vi "Monitor temp.vi"(8 "error in (no error)":errorcluster, 10 "Address":dbl=1.0, 11 "VISA resource name (IN)":refnum<visa-resource-name>) -> (0 "error out":errorcluster, 2 "Recevied Temp.  data":dbl, 3 "VISA resource name (OUT)":refnum<visa-resource-name>)   [LabVIEW 2010, in "Yudian AI508.lvlib"]
doc: "Use this template to build a VI to use as a subVI."
uses:
  <instrlib>/Yudian AI508/Yudian AI508.lvlib
panel:
  out "Recieved Raw Data":string
  out "Data buffer":string
  out "Digital shift":i32
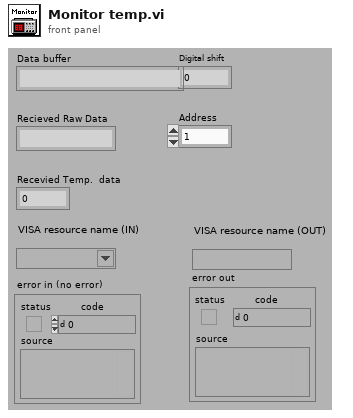
[diagram p1: front panel]
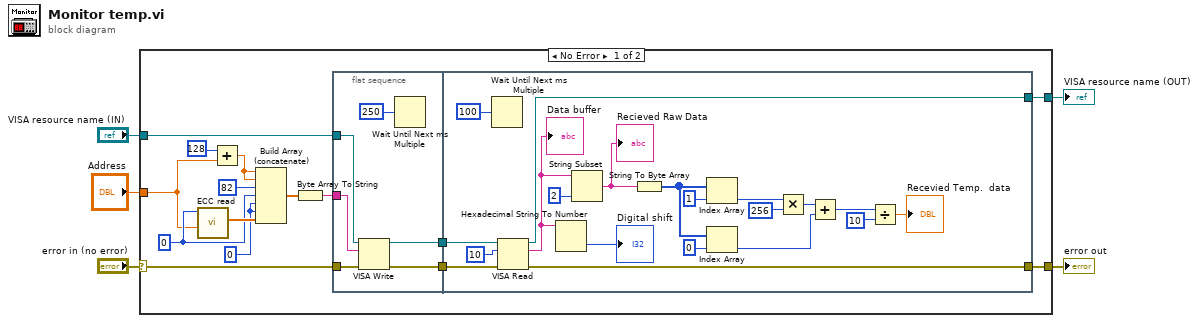
[diagram p0: block diagram]
diagram:
  n1 = case shown="No Error" "error in (no error)" {
    selector: "error in (no error)" -> [w20 w48]
    tunnel: [w16 w48] -> w5
    tunnel: [w17 w47] -> w4
    tunnel: "VISA resource name (IN)" -> [w15 w47]
    tunnel: "Address" -> [w7 _]
    frame No Error {
      w8 = 0
      w9 = 0
      n2 = call <instrlib>:"ECC read.vi"("Address"=w7, "Parameter code"=w8) -> ("Data array"=w10:dbl[])  [unwired: 9 in]
      n3 = Add(x=128, y=w7) -> (x+y=w14:dbl)
      n4 = Build Array (concatenate)(w14, w14, 82, w8, w9, w9, w10) -> (w11:dbl[])
      n5 = Byte Array To String(unsigned byte array=w11) -> (string=w6:string)
      n6 = flat-sequence {
        tunnel: w20 -> [w26]
        tunnel: [w25] -> w19
        tunnel: [w24] -> w18
        tunnel: w15 -> [w22]
        tunnel: w6 -> [w21]
        tunnel: w19 -> [w32]
        tunnel: w18 -> [w31]
        tunnel: [w29] -> w17
        tunnel: [w28] -> w16
        frame #0 {
          n7 = VISA Write(VISA resource name=w22, write buffer=w21, error in (no error)=w26) -> (VISA resource name out=w24:refnum<visa-resource-name>, error out=w25:errorcluster)  [unwired: 1 out]
          n8 = Wait Until Next ms Multiple(millisecond multiple=250) -> ()  [unwired: 1 out]
        }
        frame #1 {
          n9 = Wait Until Next ms Multiple(millisecond multiple=100) -> ()  [unwired: 1 out]
          n10 = VISA Read(VISA resource name=w31, byte count=u32 10 ("字节总数"), error in (no error)=w32) -> (VISA resource name out=w29:refnum<visa-resource-name>, read buffer=w34:string, error out=w28:errorcluster)  [unwired: 1 out]
          "Data buffer" <- w34
          n11 = Hexadecimal String To Number(string=w34) -> (number=→"Digital shift":u32)  [unwired: 3 out]
          n12 = String Subset(string=w34, length (rest)=2 ("length (rest)")) -> (substring=w44:string)  [unwired: 1 out]
          "Recieved Raw Data" <- w44
          n13 = String To Byte Array(string=w44) -> (unsigned byte array=w42:u8[])
          n14 = Index Array(array=w42, index=1) -> (element=w41:u8)
          n15 = Index Array(array=w42, index=0) -> (element=w38:u8)
          n16 = Multiply(x=w41, y=u16 256) -> (x*y=w39:u16)
          n17 = Add(x=w39, y=w38) -> (x+y=w37:u16)
          n18 = Divide(x=w37, y=u16 10) -> (x/y=→"Recevied Temp.  data":dbl)
        }
      }
    }
    frame Error {
    }
  }
  "error out" <- w5
  "VISA resource name (OUT)" <- w4
